vi "Acquire Waveform (simulated).vi"(8 "error in (no error)":errorcluster, 10 "channel #":i32, 11 "# points":i32=20) -> (0 "error out":errorcluster, 3 "waveform output":waveform(dbl))   [LabVIEW 2023]
doc: "This VI demonstrates how to create a waveform data type. The values are randomly generated for demonstration purposes."
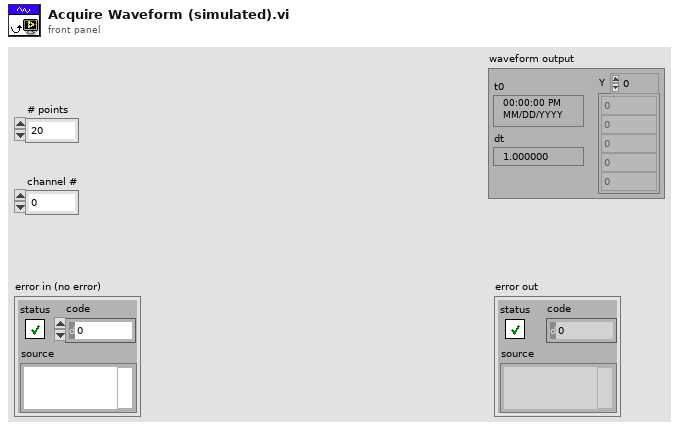
[diagram p1: front panel]
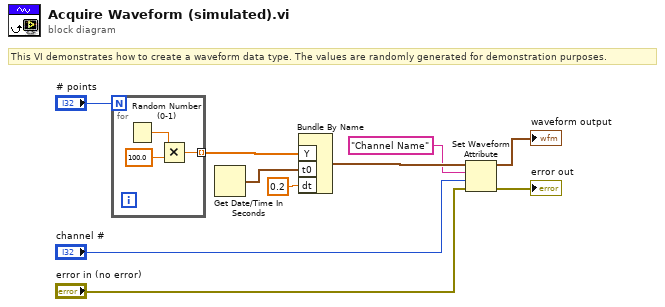
[diagram p0: block diagram]
diagram:
  # "This VI demonstrates how to create a waveform data type. The values are randomly generated for demonstration purposes."
  n1 = for {
    N: "# points" -> [_]
    tunnel: [w11] -> w9 mode=indexing
    n2 = Random Number (0-1)() -> (number: 0 to 1=w12:dbl)
    n3 = Multiply(x=w12, y=100.0) -> (x*y=w11:dbl)
  }
  n4 = Get Date/Time In Seconds() -> (seconds since 1Jan1904=w3:timestamp)
  n5 = Bundle By Name("Y"=w9, "t0"=w3, "dt"=0.2) -> (w8:waveform(dbl))  [unwired: 1 out]
  n6 = Set Waveform Attribute(4:"error in (no error)", 5:"channel #", 6:"Channel Name" ("Channel Name"), 7:w8) -> (0:→"error out":errorcluster, 3:→"waveform output":waveform(dbl))  [unwired: 1 out]
